vi "Timing_Module.vi"(7 "Command":T1, 8 "error in (no error)":errorcluster, 9 "Time In":dbl) -> (0 "error out":errorcluster, 1 "Elapsed Out":dbl, 2 "Time Elapsed":bool)   [LabVIEW 2013]
uses:
  Timing_Module Control.ctl
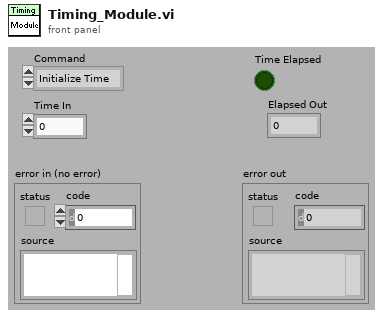
[diagram p1: front panel]
types:
  T1 = typedef "Timing_Module Control.ctl" = enum16{"Initialize Time", "Check Time"}
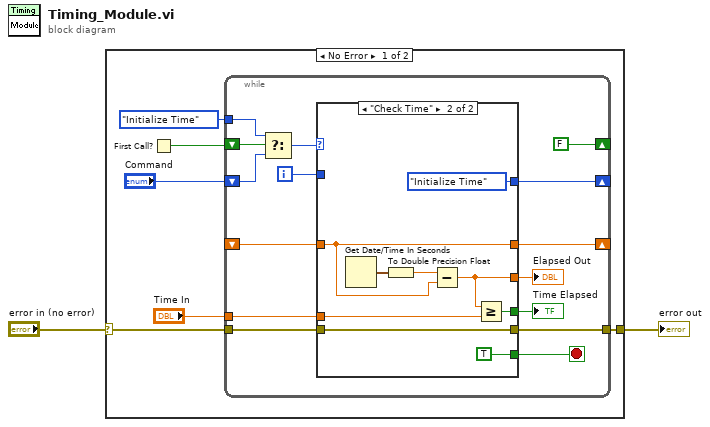
[diagram p0: block diagram]
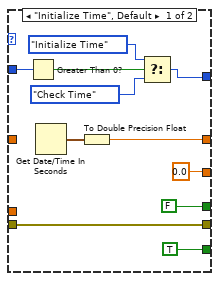
[diagram p2: hidden frame]
diagram:
  n1 = case shown="No Error" "error in (no error)" {
    selector: "error in (no error)" -> [w8 w44]
    tunnel: [w7 w44] -> w1
    frame No Error {
      n2 = First Call?() -> (First Call?: T/F=w5:bool)
      n3 = while {
        tunnel: w8 -> [w15]
        tunnel: [w14] -> w7
        shift-right: [FALSE ("First Call?: T/F")] -> _
        shift-left: w5 -> [w23]
        shift-right: [w18] -> _
        shift-left: "Command" -> [w21]
        tunnel: Timing_Module_Control."Initialize Time" ("Command") -> [w22]
        shift-right: [w16] -> _
        shift-left: _ -> [w9]
        tunnel: "Time In" -> [w11]
        i -> [w19]
        stop <- w10 stop-if-true
        n4 = Select(t=w22, s=w23, f=w21) -> (s? t:f=w20:T1)
        n5 = case shown="\"Check Time\"" w20 {
          tunnel: w19 -> [w34 _]
          tunnel: [w30 Timing_Module_Control."Initialize Time" ("Command")] -> w18
          tunnel: [w28 w36] -> w16
          tunnel: w15 -> [w27 w39]
          tunnel: [w27 w39] -> w14
          tunnel: [0.0 ("Elapsed Out") w35] -> w13
          tunnel: [FALSE ("First Call?: T/F") w38] -> w12
          tunnel: w11 -> [_ w37]
          tunnel: [TRUE ("First Call?: T/F") TRUE ("First Call?: T/F")] -> w10
          tunnel: w9 -> [_ w36]
          frame "Initialize Time", Default {
            n6 = Greater Than 0?(x=w34) -> (x > 0?=w31:bool)
            n7 = Get Date/Time In Seconds() -> (seconds since 1Jan1904=w29:timestamp)
            n8 = To Double Precision Float(number=w29) -> (double precision float=w28:dbl)
            n9 = Select(t=Timing_Module_Control."Initialize Time" ("Command"), s=w31, f=Timing_Module_Control."Check Time" ("Command")) -> (s? t:f=w30:T1)
          }
          frame "Check Time" {
            n10 = Get Date/Time In Seconds() -> (seconds since 1Jan1904=w41:timestamp)
            n11 = To Double Precision Float(number=w41) -> (double precision float=w40:dbl)
            n12 = Subtract(x=w40, y=w36) -> (x-y=w35:dbl)
            n13 = Greater Or Equal?(x=w35, y=w37) -> (x >= y?=w38:bool)
          }
        }
        "Elapsed Out" <- w13
        "Time Elapsed" <- w12
      }
    }
    frame Error {
    }
  }
  "error out" <- w1
